vi "StartListeningTask.vi"(8 "error in (no error)":errorcluster) -> (0 "error out":errorcluster)   [LabVIEW 2020, in "UmlEditor.lvclass"]
uses:
  <resource>/Framework/Providers/Open_GDS/UML/UmlEditor_class/UmlEditor.lvclass
  <resource>/Framework/Providers/Open_GDS/UML/UmlEditor_class/private/ListeningTask.vi
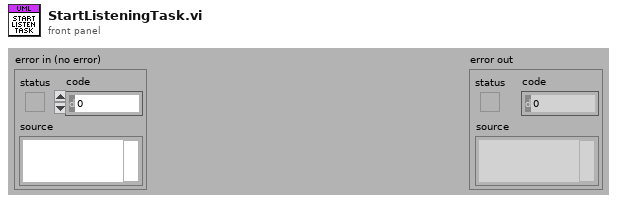
[diagram p1: front panel]
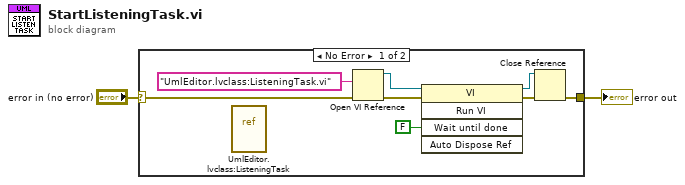
[diagram p0: block diagram]
diagram:
  n1 = case shown="No Error" "error in (no error)" {
    selector: "error in (no error)" -> [w10 w11]
    tunnel: [w4 w11] -> w1
    frame No Error {
      n2 = vi-ref "UmlEditor.lvclass:ListeningTask.vi"() -> ()  [unwired: 1 out]
      n3 = Open VI Reference(vi path="UmlEditor.lvclass:ListeningTask.vi", error in (no error)=w10) -> (vi reference=w8:refnum<vi>, error out=w7:errorcluster)  [unwired: 4 out]
      n4 = invoke class="VI" method="Run VI"(reference=w8, error in=w7, "Wait until done"=FALSE ("Wait Until Done")) -> (reference out=w6:refnum<vi>, error out=w5:errorcluster)  [unwired: 2 in, 3 out]
      n5 = Close Reference(reference=w6, error in (no error)=w5) -> (error out=w4:errorcluster)
    }
    frame Error {
    }
  }
  "error out" <- w1
